vi "Facade.vi"(0 "Data In":T4, 2 "Display State In":T2, 3 "Container State":T3) -> (6 "Data Out":T4, 7 "Display State Out":T2, 8 "Action":T1)   [LabVIEW 2020, in "DiskSpaceMonitor.xctl"]
uses:
  DiskSpaceMonitor.xctl
  Data.vi
  <vilib>/_xctls/Container State.ctl
  State.vi
  <vilib>/_xctls/Action.ctl
  <vilib>/_xctls/XControlSupport.lvlib
panel:
  out "D space":dbl(slide) caption="D: 2TB free of 2TB" scale=0.0..1.0
  out "C space":dbl(slide) caption="C: 2TB free of 2TB" scale=0.0..1.0
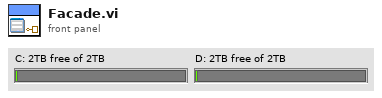
[diagram p1: front panel]
types:
  T1 = typedef "XControlSupport.lvlib/Action.ctl" = cluster{"Data Changed?":bool, "State Changed?":bool, "Action Name":string}
  T2 = typedef "DiskSpaceMonitor.xctl/State.vi" = cluster{"Numeric":dbl}
  T3 = typedef "XControlSupport.lvlib/Container State.ctl" = cluster{"Indicator?":bool, "Run Mode?":bool, " Refnum":refnum<vi>}
  T4 = typedef "DiskSpaceMonitor.xctl/Data.vi" = dbl
  T5 = typedef "LVRectTypeDef.ctl" = cluster{"Left":i16, "Top":i16, "Right":i16, "Bottom":i16}
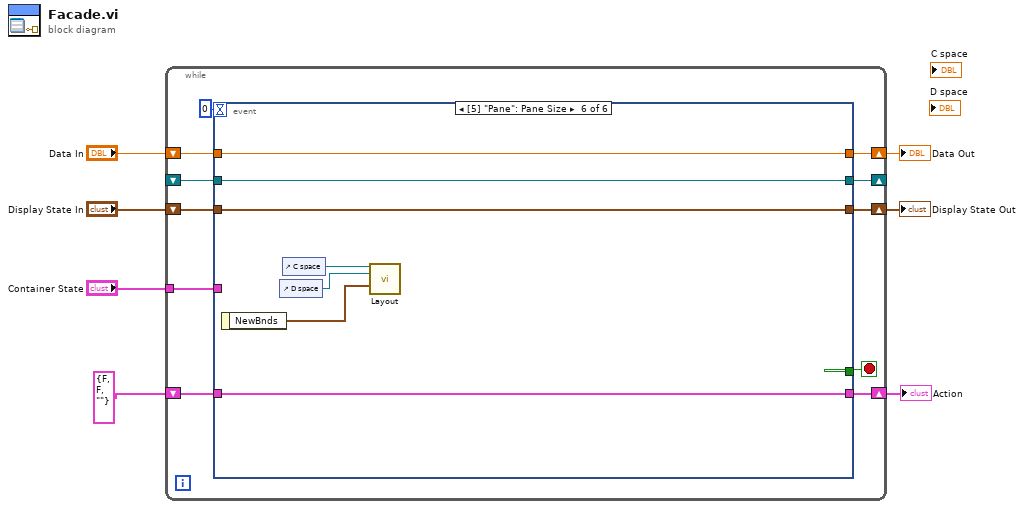
[diagram p0: block diagram]
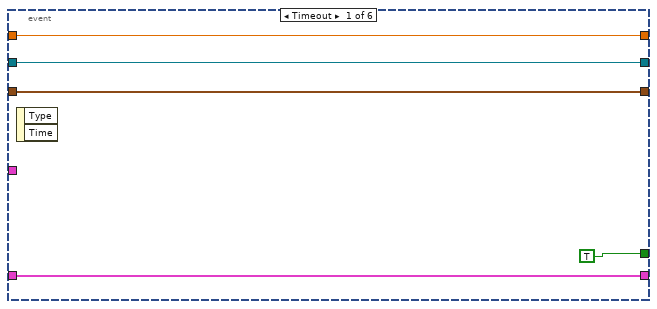
[diagram p2: hidden frame]
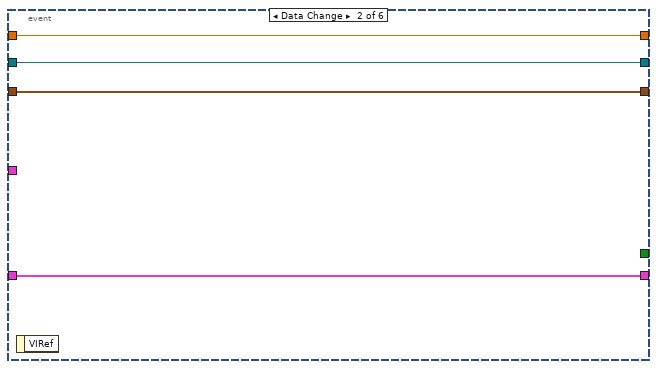
[diagram p3: hidden frame]
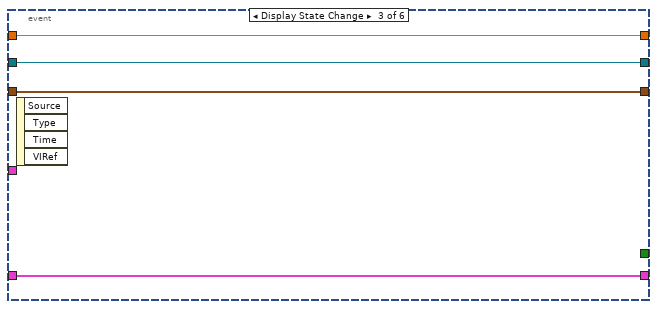
[diagram p4: hidden frame]
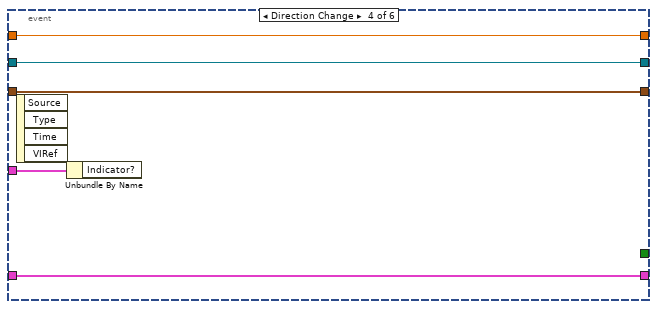
[diagram p5: hidden frame]
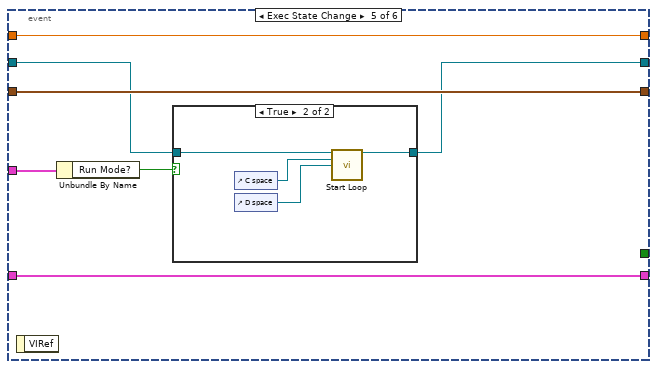
[diagram p6: hidden frame]
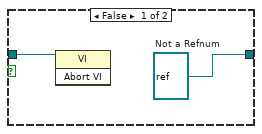
[diagram p7: hidden frame]
diagram:
  n1 = while {
    shift-right: [w17] -> w4
    shift-left: "Display State In" -> [w18]
    tunnel: "Container State" -> [w14]
    shift-right: [w12] -> w7
    shift-left: "Data In" -> [w13]
    shift-right: [w10] -> w2
    shift-left: T1 {"Data Changed?"=FALSE, "State Changed?"=FALSE, "Action Name"=""} ("Action") -> [w11]
    shift-right: [w9] -> _
    shift-left: _ -> [w8]
    stop <- w16 stop-if-true
    n2 = event shown="[5] \"Pane\": Pane Size" {
      selector: _ -> [_ _ _ _ _ _]
      dyn-events: _ -> [_ _ _ _ _ _]
      timeout: 0 -> [_ _ _ _ _ _]
      tunnel: w18 -> [w21 w26 w31 w35 w42 w56]
      tunnel: [w21 w26 w31 w35 w42 w56] -> w17
      tunnel: [TRUE _ _ _ _ _] -> w16
      tunnel: w14 -> [_ _ _ w36 w43 _]
      tunnel: w13 -> [w20 w27 w30 w34 w41 w55]
      tunnel: [w20 w27 w30 w34 w41 w55] -> w12
      tunnel: [w22 w25 w29 w33 w40 w54] -> w10
      tunnel: w11 -> [w22 w25 w29 w33 w40 w54]
      tunnel: [w19 w24 w28 w32 w38 w53] -> w9
      tunnel: w8 -> [w19 w24 w28 w32 w37 w53]
      event Timeout {
        n3 = event-data() -> ()  [unwired: 1 in, 2 out]
      }
      event Data Change {
        n4 = event-data() -> ()  [unwired: 1 in, 1 out]
      }
      event Display State Change {
        n5 = event-data() -> ()  [unwired: 1 in, 4 out]
      }
      event Direction Change {
        n6 = event-data() -> ()  [unwired: 1 in, 4 out]
        n7 = Unbundle By Name(w36) -> ()  [unwired: 1 out]
      }
      event Exec State Change {
        n8 = event-data() -> ()  [unwired: 1 in, 1 out]
        n9 = Unbundle By Name(w43) -> ("Run Mode?"=w39:bool)
        n10 = case shown="True" w39 {
          tunnel: [w45 w49] -> w38
          tunnel: w37 -> [w44 w48]
          frame False {
            w45 = refnum<vi> refnum  # Not a Refnum
            n11 = invoke class="VI" method="Abort VI"(reference=w44) -> ()  [unwired: 2 in, 3 out]
          }
          frame True {
            n12 = control-ref of="C space"() -> (w47:refnum<vi>)
            n13 = control-ref of="D space"() -> (w46:refnum<vi>)
            n14 = call "Start Loop.vi"("vi reference in"=w48, "C space"=w47, "D space"=w46) -> ("vi reference out"=w49:refnum<vi>)  [unwired: 11 in, 1 out]
          }
        }
      }
      event Pane Size {
        n15 = event-data() -> ("NewBnds"=w52:T5)  [unwired: 1 in]
        n16 = control-ref of="D space"() -> (w50:refnum<vi>)
        n17 = control-ref of="C space"() -> (w51:refnum<vi>)
        n18 = call "Layout.vi"("Slide in"=w51, "D space"=w50, "NewBnds"=w52) -> ()  [unwired: 13 in]
      }
    }
  }
  "Display State Out" <- w4
  "Data Out" <- w7
  "Action" <- w2
